vi "Color Pattern Matching.vi"() -> ()   [LabVIEW 2018]
doc: "This example shows how to use the color pattern matching tools in NI Vision.\n\nYou use color pattern matching to locate known reference or fiducial patterns in an image quickly. Pattern matching is the key to many applications. Color pattern matching can provide your application with information about the presence or absence, number, and location of the model within an image.\n\nYou use color pattern matching in the following three general applications areas:\n\n* Alignment -- Determine the position and orientation of a known object by locating features. You use the features as points of reference on the object.\n\n* Gauging -- Measure lengths, diameters, angles, and other critical dimensions. If the measurements fall outside of set tolerance levels, the component is rejected. You sometimes use gauging in-line with the manufacturing process and off-line. If you make the measurements off-line, a sample of components is used to determine the quality of a lot or batch of manufactured components.\n\n* Inspection -- Detect simple flaws, such as missing parts or unreadable printing."
uses:
  <vilib>/vision/NI_Vision_Development_Module.lvlib
panel:
  out "Number of Matches":i32
  out "Results":T1(array[cluster]) {"Position"."Y" format="%.2f"; "Position"."X" format="%.2f"}
  in  "Max # of Matches":i32=5
  in  "Minimum Score":sgl=700.0
  out "Template":T2(plugin-control)
  in  "Stop":bool
  out "Image":T2(plugin-control)
  # "Overview: Demonstrates how to perform Color Pattern Matching using two steps that include learning the color pattern template defined by a Region of Interest (ROI) and then matching the learned template in the image.\nRequirements: Vision Development Software.\nInstructions:\n1. Run the VI.\n2. Draw a ROI in the image to define the template. The learned template is displayed in the Template display and the match results are overlaid on the Image display."
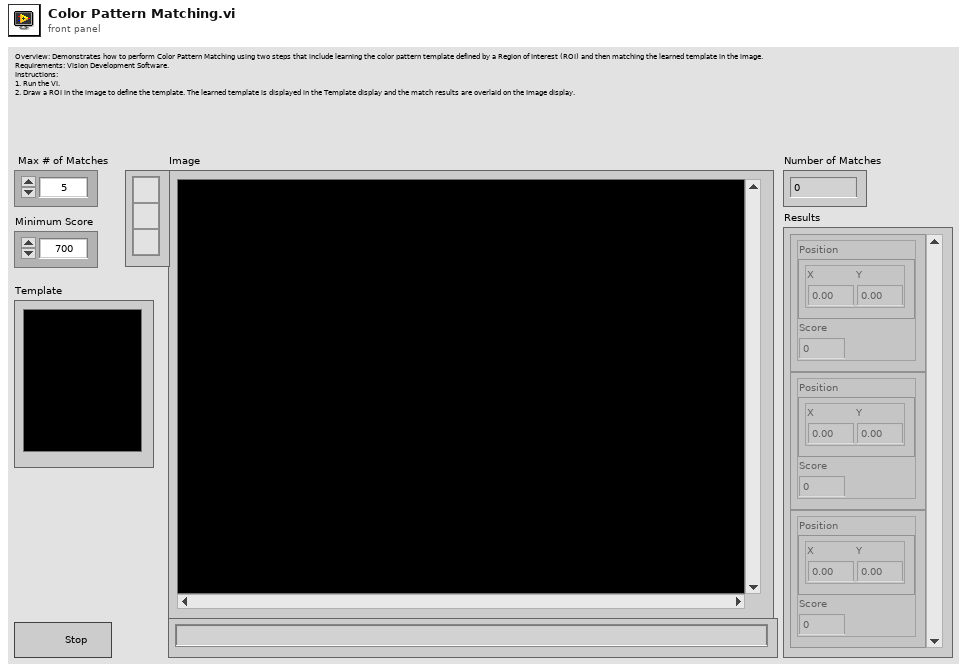
[diagram p1: front panel]
types:
  T1 = cluster{"Position":cluster{"X":dbl, "Y":dbl}, "Score":dbl}[]
  T2 = typedef "IMAQ Image.ctl" = refnum<image>
  T3 = typedef "Image Type" = u32
  T4 = typedef "IMAQ Rectangle" = cluster{"Left":i32, "Top":i32, "Right":i32, "Bottom":i32, "Rotation":dbl}
  T5 = typedef "ROI Descriptor" = cluster{"Global Rectangle":i32[], "Contours":cluster{"ID":enum32{"External", "Internal"}, "Type":u32, "Coordinates":i32[]}[]}
  T6 = cluster{"Max # of Matches":i32, "Minimum Score":sgl}
  T7 = cluster{"Position":cluster{"x":sgl, "y":sgl}, "Angle":sgl, "Scale":sgl, "Score":sgl, "Bounding Box":cluster{"x":sgl, "y":sgl}[]}[]
  T8 = cluster{"Position":cluster{"x":sgl, "y":sgl}, "Score":sgl}
  T9 = cluster{i32[], cluster{"Contour Type":u32, "ROI Type":u32, i32[]}[]}
  T10 = cluster{"Global Rectangle":i32[], "Contours":cluster{"Contour Type":u32, "ROI Type":u32, "Points":i32[]}[]}
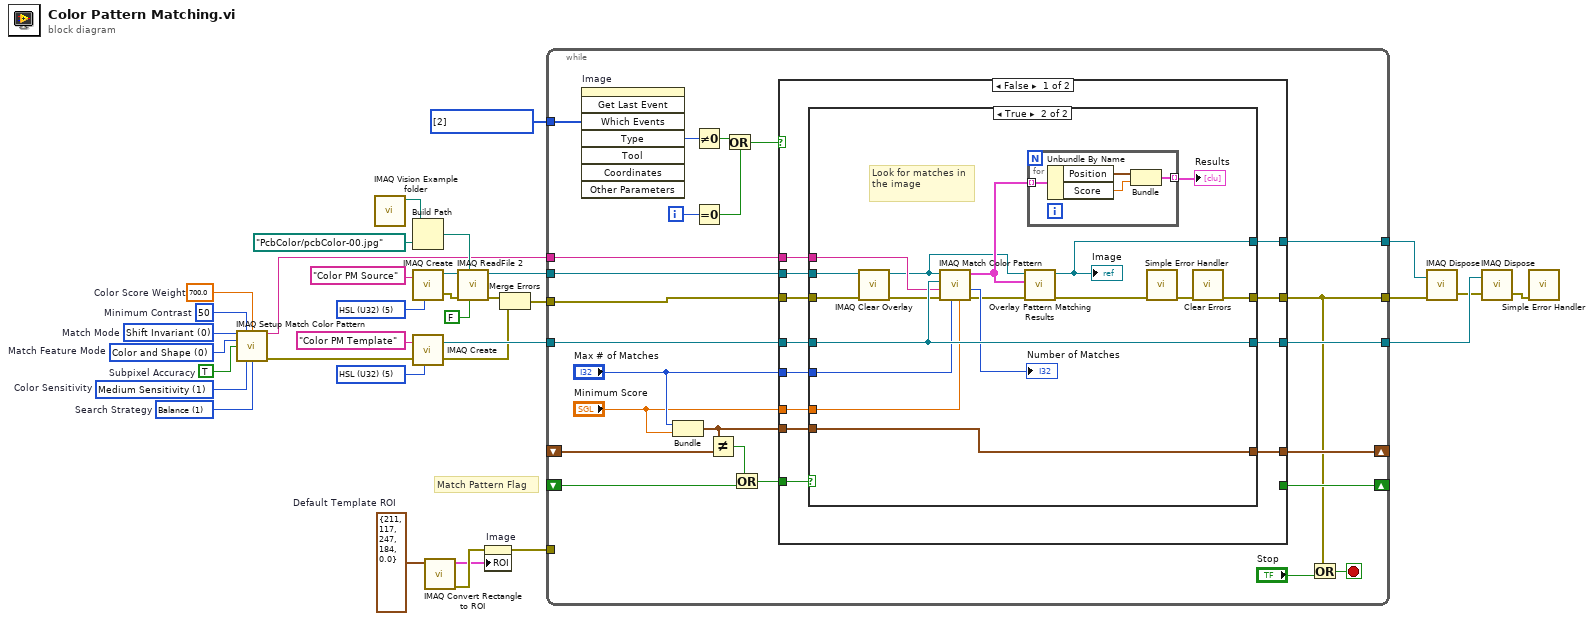
[diagram p0: block diagram]
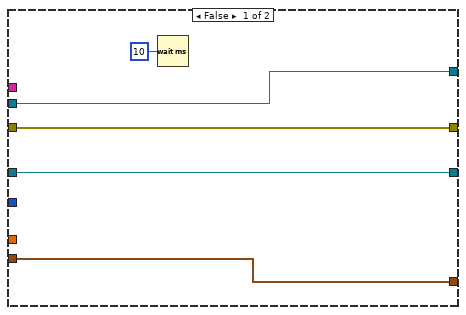
[diagram p2: hidden frame]
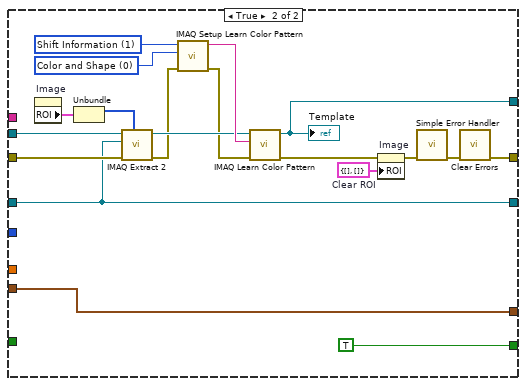
[diagram p3: hidden frame]
diagram:
  w2 = TRUE  # Subpixel Accuracy
  w10 = u32 0 items=["Color and Shape", "Color", "Shape"]  # Match Feature Mode
  w9 = u32 1 items=["Conservative", "Balance", "Aggressive", "Very Aggressive"]  # Search Strategy
  w8 = 50  # Minimum Contrast
  w7 = sgl 700.0  # Color Score Weight
  w6 = u32 1 items=["Low Sensitivity", "Medium Sensitivity", "High Sensitivity"]  # Color Sensitivity
  w5 = u32 0 items=["Shift Invariant", "Rotation Invariant"]  # Match Mode
  w22 = T3 5 items=["Grayscale (U8)", "Grayscale (I16)", "Grayscale (SGL)", "Complex (CSG)", "RGB (U32)", "HSL (U32)", "RGB (U64)", "Grayscale (U16)"] ("Image Type")
  w23 = T3 5 items=["Grayscale (U8)", "Grayscale (I16)", "Grayscale (SGL)", "Complex (CSG)", "RGB (U32)", "HSL (U32)", "RGB (U64)", "Grayscale (U16)"] ("Image Type")
  w28 = i32[] [2] items=["No Event"=0, "Click Event"=1, "Draw Event"=2, "Size Event"=4, "Scroll Event"=5, "Double Click Event"=8] ("Which Events")
  w30 = T4 {"Left"=211, "Top"=117, "Right"=247, "Bottom"=184, "Rotation"=0.0}  # Default Template ROI
  # "Match Pattern Flag"
  n1 = call "IMAQ Setup Match Color Pattern"("Match Mode"=w5, "Minimum Contrast"=w8, "Color Score Weight"=w7, "Match Feature Mode"=w10, "Subpixel Accuracy"=w2, "Color Sensitivity"=w6, "Search Strategy"=w9) -> ("Match Color Pattern Setup Data"=w3:string, "error out"=w4:errorcluster)  [unwired: 7 in]
  n2 = call "IMAQ Vision Example folder.vi"() -> ("Example Image Path"=w33:path)  [unwired: 11 in]
  n3 = Build Path(base path=w33, name or relative path=path "PcbColor/pcbColor-00.jpg") -> (appended path=w29:path)
  n4 = call "IMAQ Create"("Image Name"="Color PM Source", "Image Type"=w23) -> ("New Image"=w14:T2, "error out"=w19:errorcluster)  [unwired: 3 in]
  n5 = call "IMAQ Create"("Image Name"="Color PM Template", "Image Type"=w22, "error in (no error)"=w4) -> ("New Image"=w27:T2, "error out"=w16:errorcluster)  [unwired: 2 in]
  n6 = call "IMAQ Convert Rectangle to ROI"("Rectangle"=w30) -> ("error out"=w18:errorcluster, "ROI Descriptor"=w12:T5)  [unwired: 8 in]
  n7 = call "IMAQ ReadFile 2"("Use File Path Image Type"=FALSE, "File Path"=w29, "error in (no error)"=w19, "Image"=w14) -> ("error out"=w17:errorcluster, "Image Out"=w13:T2)  [unwired: 3 in, 3 out]
  n8 = property on="Image" class="ImageControl"(error in=w18, "ROI"=w12) -> (error out=w11:errorcluster)  [unwired: 1 in, 1 out]
  n9 = Merge Errors(w17, w16) -> (w15:errorcluster)
  n10 = while {
    tunnel: w13 -> [w48]
    tunnel: w28 -> [w58]
    tunnel: w27 -> [w47]
    tunnel: w15 -> [w52]
    shift-right: [w46] -> _
    shift-left: _ -> [w39]
    shift-right: [w51] -> _
    shift-left: _ -> [w50]
    tunnel: [w44] -> w26
    tunnel: [w45] -> w25
    tunnel: [w37] -> w24
    tunnel: w11 -> [_]
    tunnel: w3 -> [w41]
    i -> [w55]
    stop <- w35 stop-if-true
    n11 = invoke on="Image" class="ImageControl" method="Get Last Event"("Which Events"=w58) -> ("Type"=w57:i32)  [unwired: 7 in, 7 out]
    n12 = Bundle("Max # of Matches"="Max # of Matches", "Minimum Score"="Minimum Score") -> (w40:T6)  [unwired: 1 in]
    n13 = Not Equal To 0?(x=w57) -> (x != 0?=w56:bool)
    n14 = Equal To 0?(x=w55) -> (x = 0?=w54:bool)
    n15 = Not Equal?(x=w40, y=w39) -> (x != y?=w38:bool)
    n16 = Or(x=w56, y=w54) -> (x .or. y?=w53:bool)
    n17 = Or(x=w38, y=w50) -> (x .or. y?=w49:bool)
    n18 = case shown="False" w53 {
      tunnel: w48 -> [w68 w106]
      tunnel: w52 -> [w67 w105]
      tunnel: w47 -> [w66 w98]
      tunnel: [_ TRUE] -> w51
      tunnel: w49 -> [w70 _]
      tunnel: w40 -> [w69 w97]
      tunnel: [w65 w101] -> w37
      tunnel: [w64 w97] -> w46
      tunnel: [w63 w98] -> w45
      tunnel: [w62 w99] -> w44
      tunnel: "Max # of Matches" -> [w61 _]
      tunnel: "Minimum Score" -> [w60 _]
      tunnel: w41 -> [w59 _]
      frame False {
        n19 = case shown="True" w70 {
          tunnel: w69 -> [w73 w89]
          tunnel: w68 -> [w71 w92]
          tunnel: w67 -> [w75 w91]
          tunnel: w66 -> [w72 w90]
          tunnel: [w75 w87] -> w65
          tunnel: [w73 w89] -> w64
          tunnel: [w72 w90] -> w63
          tunnel: [w71 w77] -> w62
          tunnel: w61 -> [_ w85]
          tunnel: w60 -> [_ w84]
          tunnel: w59 -> [_ w83]
          frame False {
            n20 = Wait (ms)(milliseconds to wait=u32 10) -> ()  [unwired: 1 out]
          }
          frame True {
            # "Look for matches in the image"
            n21 = call "IMAQ Clear Overlay"("error in (no error)"=w91, "Image"=w92) -> ("error out"=w86:errorcluster, "Image Out"=w76:T2)  [unwired: 8 in]
            n22 = call "IMAQ Match Color Pattern"("Minimum Match Score"=w84, "Number of Matches Requested"=w85, "error in (no error)"=w86, "Match Color Pattern Setup Data"=w83, "Template Image"=w90, "Image"=w76) -> ("error out"=w80:errorcluster, "Number of Matches"=→"Number of Matches":i32, "Matches"=w79:T7)  [unwired: 3 in]
            n23 = call "Overlay Pattern Matching Results.vi"("error in"=w80, "Matches"=w79, "Image"=w76) -> ("error out"=w78:errorcluster, "Image Out"=w77:T2)  [unwired: 7 in]
            "Image" <- w77
            n24 = for {
              tunnel: w79 -> [w96] mode=indexing
              tunnel: [w93] -> w82 mode=indexing
              n25 = Unbundle By Name(w96) -> ("Position"=w95:cluster{"x":sgl, "y":sgl}, "Score"=w94:sgl)
              n26 = Bundle("Position"=w95, "Score"=w94) -> (w93:T8)  [unwired: 1 in]
            }
            "Results" <- w82
            n27 = call <vilib>:"Simple Error Handler.vi"("error in (no error)"=w78) -> ("error out"=w88:errorcluster)  [unwired: 4 in, 4 out]
            n28 = call <vilib>:"Clear Errors.vi"("error in (no error)"=w88) -> ("error out"=w87:errorcluster)  [unwired: 5 in, 1 out]
          }
        }
      }
      frame True {
        w103 = u32 0 items=["Color and Shape", "Color", "Shape "] ("Feature Mode")
        w107 = u32 1 items=["All", "Shift Information", "Rotation Information"] ("Learn Mode")
        w108 = T9 {[], []}  # Clear ROI
        n29 = property on="Image" class="ImageControl"() -> ("ROI"=w110:T10)  [unwired: 2 in, 2 out]
        n30 = Unbundle(w110) -> ("Global Rectangle"=w115:i32[])  [unwired: 1 out]
        n31 = call "IMAQ Extract 2"("Optional Rectangle"=w115, "error in (no error)"=w105, "Image Dst"=w98, "Image Src"=w106) -> ("error out"=w112:errorcluster, "Image Dst Out"=w113:T2)  [unwired: 6 in]
        n32 = call "IMAQ Setup Learn Color Pattern"("error in (no error)"=w112, "Feature Mode"=w103, "Learn Mode"=w107) -> ("error out"=w111:errorcluster, "Learn Color Pattern Setup Data"=w114:string)  [unwired: 7 in]
        n33 = call "IMAQ Learn Color Pattern"("error in (no error)"=w111, "Learn Color Pattern Setup Data"=w114, "Image"=w113) -> ("error out"=w100:errorcluster, "Template Image Out"=w99:T2)  [unwired: 7 in]
        "Template" <- w99
        n34 = property on="Image" class="ImageControl"(error in=w100, "ROI"=w108) -> (error out=w109:errorcluster)  [unwired: 1 in, 1 out]
        n35 = call <vilib>:"Simple Error Handler.vi"("error in (no error)"=w109) -> ("error out"=w102:errorcluster)  [unwired: 4 in, 4 out]
        n36 = call <vilib>:"Clear Errors.vi"("error in (no error)"=w102) -> ("error out"=w101:errorcluster)  [unwired: 5 in, 1 out]
      }
    }
    n37 = Or(x=w37, y="Stop") -> (x .or. y?=w35:bool)
  }
  n38 = call "IMAQ Dispose"("Image"=w26, "error in (no error)"=w24) -> ("error out"=w21:errorcluster)  [unwired: 4 in]
  n39 = call "IMAQ Dispose"("Image"=w25, "error in (no error)"=w21) -> ("error out"=w20:errorcluster)  [unwired: 4 in]
  n40 = call <vilib>:"Simple Error Handler.vi"("error in (no error)"=w20) -> ()  [unwired: 4 in, 5 out]
